vi "Create FileHandler.vi"(6 "Flush Timeout (0 s)":dbl, 7 "Formatter.lvclass":refnum<class "Formatter.lvclass">, 8 "error in":errorcluster, 9 "Level":T1, 10 "Name":string, 11 "Filepath":path) -> (0 "error out":errorcluster, 3 "FileHandler out":refnum<class "FileHandler.lvclass">)   [LabVIEW 2024, in "hse-logger.lvlib" / "FileHandler.lvclass"]
doc: "Creates and initializes a new FileHandler object.\n\n____\nHAMPEL SOFTWARE ENGINEERING v2.2.2 (2025-01-16 15:41)"
uses:
  <vilib>/Hampel Software Engineering/HSE Logger/Handler/FileHandler/FileHandler.lvclass
  <vilib>/Hampel Software Engineering/HSE Logger/LogLevel.ctl
  <vilib>/Hampel Software Engineering/HSE Logger/Formatter/Formatter.lvclass
  <vilib>/Hampel Software Engineering/HSE Logger/hse-logger.lvlib
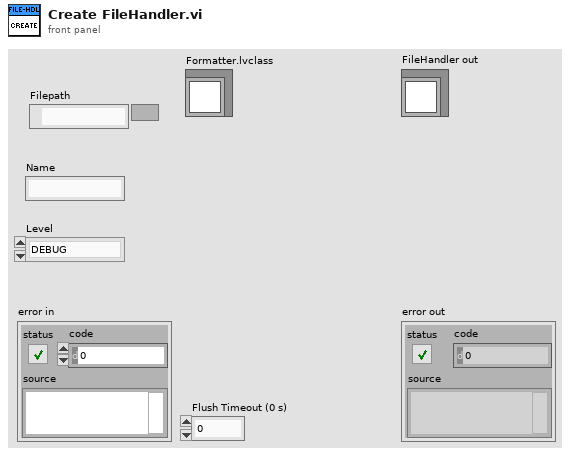
[diagram p1: front panel]
types:
  T1 = typedef "hse-logger.lvlib/LogLevel.ctl" = enum16{"DEBUG", "INFO", "WARNING", "ERROR", "CRITICAL"}
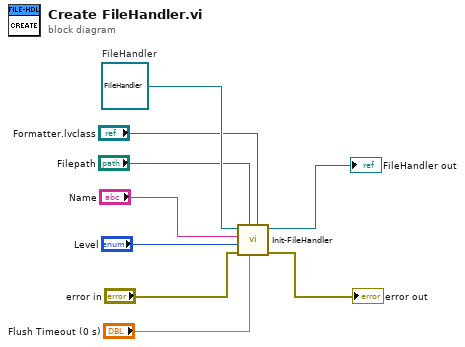
[diagram p0: block diagram]
diagram:
  w9 = refnum<class "FileHandler.lvclass"> refnum  # FileHandler
  n1 = call-dynamic "Init-FileHandler.vi"("Formatter.lvclass"="Formatter.lvclass", "Flush Timeout (5 s)"="Flush Timeout (0 s)", "Filepath"="Filepath", "error in"="error in", "Level"="Level", "Name"="Name", "FileHandler"=w9) -> ("error out"=→"error out":errorcluster, "FileHandler out"=→"FileHandler out":refnum<class "FileHandler.lvclass">)  [unwired: 3 in]
